vi "Load zero position.vi"(8 "error in (no error)":errorcluster) -> (0 "error out":errorcluster, 3 "Zero position":cluster{"M1":dbl, "M2":dbl})   [LabVIEW 2020]
uses:
  <vilib>/Utility/config.llb/NI_LVConfig.lvlib
  <vilib>/Utility/config.llb/Read Key (Double).vi
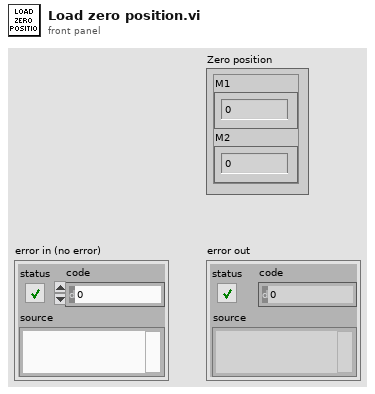
[diagram p1: front panel]
types:
  T1 = typedef "NI_LVConfig.lvlib/Config Data RefNum.ctl" = refnum<k1>
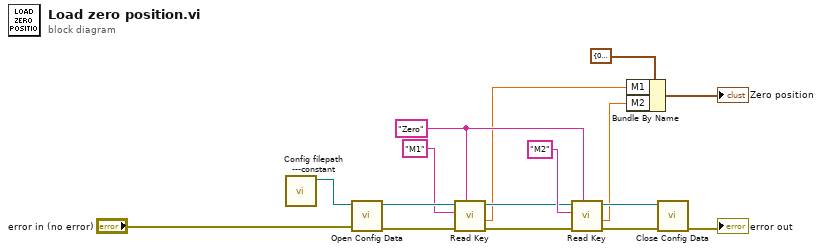
[diagram p0: block diagram]
diagram:
  w10 = "Zero" ("section")
  n1 = call "Config filepath ---constant.vi"() -> ("config file path"=w5:path)  [unwired: 11 in]
  n2 = call <vilib>:"Open Config Data.vi"("error in (no error)"="error in (no error)", "configuration file path"=w5) -> ("error out"=w15:errorcluster, "refnum"=w14:T1)  [unwired: 7 in, 1 out]
  n3 = call-poly <vilib>:"Read Key.vi"("section"=w10, "error in (no error)"=w15, "key"="M1", "refnum"=w14) -> ("error out"=w12:errorcluster, "value"=w3:dbl, "refnum out"=w6:T1)  [unwired: 4 in, 1 out]
  n4 = call-poly <vilib>:"Read Key.vi"("section"=w10, "error in (no error)"=w12, "key"="M2", "refnum"=w6) -> ("error out"=w11:errorcluster, "value"=w2:dbl, "refnum out"=w7:T1)  [unwired: 4 in, 1 out]
  n5 = Bundle By Name(cluster=cluster{"M1":dbl, "M2":dbl} {"M1"=0.0, "M2"=0.0} ("Zero position"), "M1"=w3, "M2"=w2) -> (→"Zero position":cluster{"M1":dbl, "M2":dbl})
  n6 = call <vilib>:"Close Config Data.vi"("error in (no error)"=w11, "refnum"=w7) -> ("error out"=→"error out":errorcluster)  [unwired: 8 in, 1 out]
